vi "SVFA Real and Imaginary to Magnitude and Phase.vi"   [LabVIEW 2017]
doc: "Converts spectra from rectangular components to polar components. You can display magnitude and phase information on graphs and send this information to other Spectrum Extended Measurements VIs. Wire data to the <B>real spectrum</B> and <B>imaginary spectrum</B> inputs to determine the polymorphic instance to use or manually select the instance."
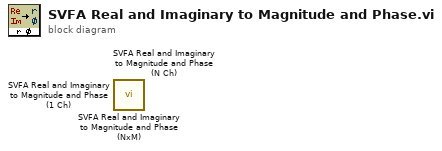
[diagram p0: block diagram]
diagram:
  n1 = call <vilib>:"SVFA Real and Imaginary to Magnitude and Phase (NxM).vi"() -> ()  [unwired: 14 in, 6 out]
  n2 = call <vilib>:"SVFA Real and Imaginary to Magnitude and Phase (N Ch).vi"() -> ()  [unwired: 14 in, 6 out]
  n3 = call <vilib>:"SVFA Real and Imaginary to Magnitude and Phase (1 Ch).vi"() -> ()  [unwired: 14 in, 6 out]
